vi "Combine Arrays (Robot).vi"(1 "Variable Names":string[](array[string]), 2 "Array of Numbers":dbl[](array[numeric])) -> (0 "Constants":cluster{"output string":string, dbl}[](array[cluster]))   [LabVIEW 2013]
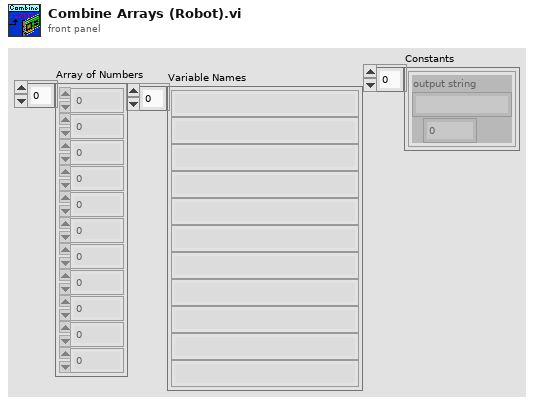
[diagram p1: front panel]
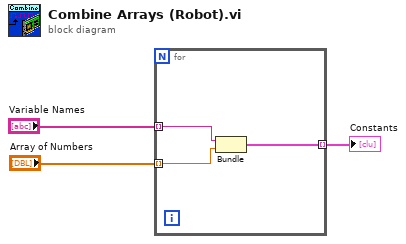
[diagram p0: block diagram]
diagram:
  n1 = for {
    tunnel: "Variable Names" -> [w6] mode=indexing
    tunnel: "Array of Numbers" -> [w5] mode=indexing
    tunnel: [w4] -> w1 mode=indexing
    n2 = Bundle("output string"=w6, w5) -> (w4:cluster{"output string":string, dbl})  [unwired: 1 in]
  }
  "Constants" <- w1
